vi "pmu_Phasors Block CFG-3 (Std 2011).vi"(0 "phasor scale factors":sgl[](array[numeric]), 1 "nominal frequency":enum16{"50 Hz", "60 Hz"}(ring), 2 "init meas data":u8[](array[numeric]), 5 "phasor angle offsets [rad]":sgl[](array[numeric]), 7 "data format":u16, 9 "measurement data":T1 {"data error" format="%02b"; "PMU time quality" format="%03b"}, 12 "analog scale factors":sgl[](array[numeric]), 13 "analog magnitude offsets":sgl[](array[numeric])) -> (4 "data block":u8[](array[numeric]) format="%x", 6 "phasor out of range":bool, 8 "freq out of range":bool, 10 "df/dt out of range":bool, 14 "analog out of range":bool)   [LabVIEW 2014, in "NI_EP_PMU.lvlib"]
doc: "This VI converts phasor data cluster to binary data block."
uses:
  <vilib>/addons/Electrical Power/PMU/NI_EP_PMU.lvlib
  <vilib>/addons/Electrical Power/PMU/Common/Controls/pmu_Measurement Data (Std 2011).ctl
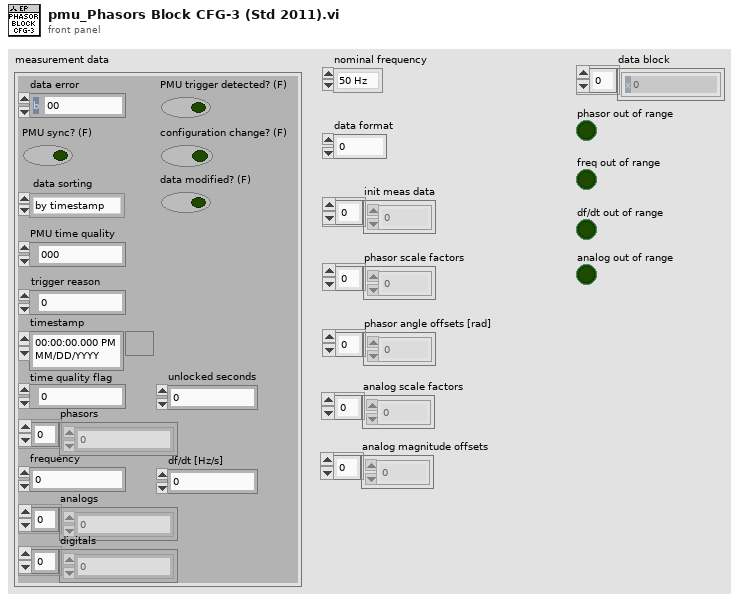
[diagram p1: front panel]
types:
  T1 = typedef "NI_EP_PMU.lvlib/pmu_Measurement Data (Std 2011).ctl" = cluster{"data error":u8, "PMU sync? (F)":bool, "data sorting":enum16{"by timestamp", "by arrival"}, "PMU trigger detected? (F)":bool, "configuration change? (F)":bool, "data modified? (F)":bool, "PMU time quality":u8, "trigger reason":u8, "timestamp":timestamp, "time quality flag":u8, "unlocked seconds":u32, "phasors":csg[], "frequency":sgl, "df/dt [Hz/s]":sgl, "analogs":sgl[], "digitals":u16[]}
  T2 = cluster{"analog scale factors":sgl[], "analog magnitude offsets":sgl[]}
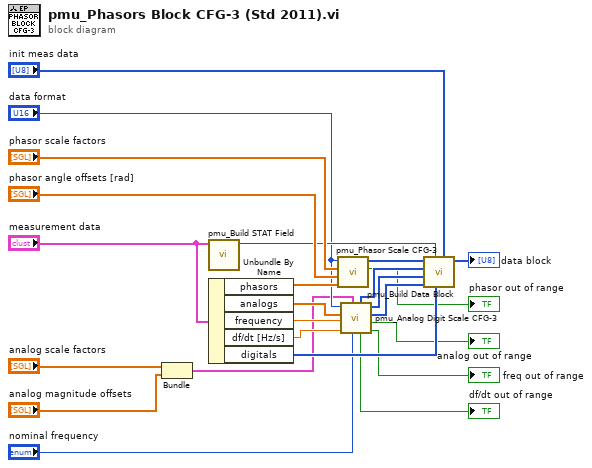
[diagram p0: block diagram]
diagram:
  n1 = Bundle("analog scale factors"="analog scale factors", "analog magnitude offsets"="analog magnitude offsets") -> (w1:T2)  [unwired: 1 in]
  n2 = call <vilib>:"pmu_Build STAT Field.vi"("measurement data"="measurement data") -> ("STAT field"=w19:u16)  [unwired: 10 in]
  n3 = Unbundle By Name("measurement data") -> ("phasors"=w21:csg[], "analogs"=w16:sgl[], "frequency"=w15:sgl, "df/dt [Hz/s]"=w14:sgl, "digitals"=w13:u16[])
  n4 = call <vilib>:"pmu_Phasor Scale CFG-3.vi"("phasors in"=w21, "phasor angle offsets [rad]"="phasor angle offsets [rad]", "phasor scale factors"="phasor scale factors", "format"="data format") -> ("phasor out of range"=→"phasor out of range":bool, "phasor byte array"=w20:u8[])  [unwired: 6 in]
  n5 = call <vilib>:"pmu_Analog Digit Scale CFG-3.vi"("nominal frequency"="nominal frequency", "analog scaling"=w1, "dfreq in"=w14, "freq in"=w15, "analogs in"=w16, "format"="data format") -> ("freq out of range"=→"freq out of range":bool, "analog out of range"=→"analog out of range":bool, "analogs byte array"=w10:u8[], "dfreq byte array"=w11:u8[], "df/dt out of range"=→"df/dt out of range":bool, "freq byte array"=w12:u8[])
  n6 = call <vilib>:"pmu_Build Data Block.vi"("init meas data"="init meas data", "digitals"=w13, "STAT field"=w19, "analogs byte array"=w10, "dfreq byte array"=w11, "freq byte array"=w12, "phasor byte array"=w20) -> ("data block"=→"data block":u8[])  [unwired: 4 in]
